vi "plotTrajectories.vi"(1 "Trajectories":sgl[][](array[numeric])) -> (0 "PlotID":i32[](array[numeric]))   [LabVIEW 2023]
uses:
  <vilib>/Math Plots/3D Math Plots/3D Scatter/3D Scatter Datatype/3D Scatter Datatype.lvclass
  <vilib>/Math Plots/3D Math Plots/3D Scatter/3D Scatter Datatype/Public/Plot Helper (Vector).vi
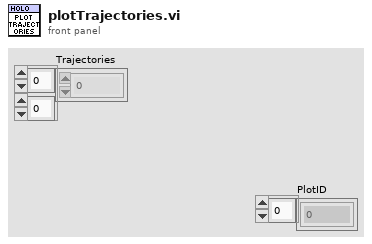
[diagram p1: front panel]
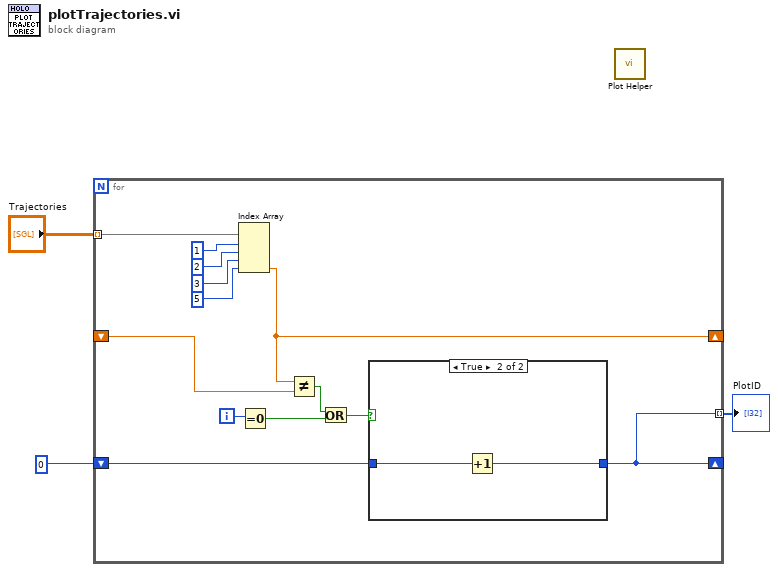
[diagram p0: block diagram]
diagram:
  n1 = for {
    tunnel: "Trajectories" -> [w16] mode=indexing
    shift-right: [w10] -> _
    shift-left: _ -> [w11]
    shift-right: [w4] -> _
    shift-left: 0 -> [w5]
    tunnel: [w4] -> w1 mode=indexing
    i -> [w7]
    n2 = Index Array(array=w16, index #1=1 ("disabled index (col)"), index #2=2 ("index (col)"), index #3=3 ("index (col)"), index #4=5 ("index (col)")) -> (element #4=w10:sgl)  [unwired: 3 out]
    n3 = Equal To 0?(x=w7) -> (x = 0?=w6:bool)
    n4 = Not Equal?(x=w10, y=w11) -> (x != y?=w9:bool)
    n5 = Or(x=w9, y=w6) -> (x .or. y?=w8:bool)
    n6 = case shown="True" w8 {
      tunnel: w5 -> [w17 w19]
      tunnel: [w17 w18] -> w4
      frame False {
      }
      frame True {
        n7 = Increment(x=w19) -> (x+1=w18:i32)
      }
    }
  }
  "PlotID" <- w1
  n8 = call-poly <vilib>:"Plot Helper.vi"() -> ()  [unwired: 6 in, 6 out]
